vi "6-3 Write.vi"() -> ()   [LabVIEW 2017]
panel:
  out "Waveform Chart":dbl(graph)
  in  "stop":bool
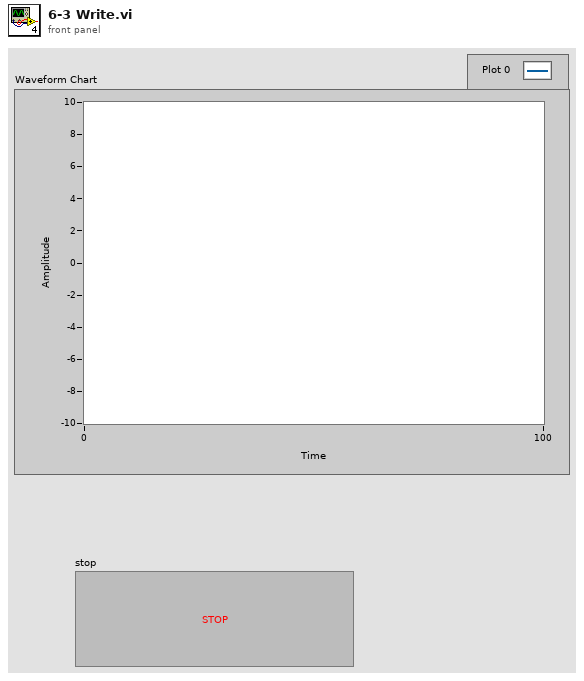
[diagram p1: front panel]
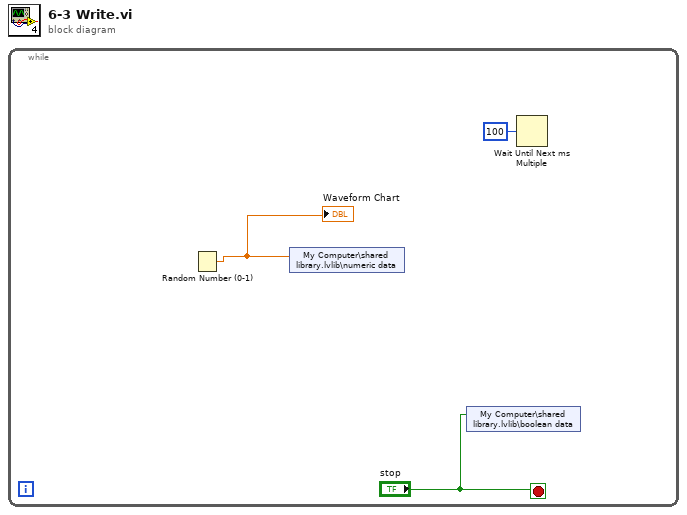
[diagram p0: block diagram]
diagram:
  n1 = while {
    stop <- "stop" stop-if-true
    n2 = Random Number (0-1)() -> (number: 0 to 1=w2:dbl)
    "Waveform Chart" <- w2
    n3 = shared-variable "My Computer\\shared library.lvlib\\numeric data"(w2) -> ()  [unwired: 1 in, 1 out]
    n4 = shared-variable "My Computer\\shared library.lvlib\\boolean data"("stop") -> ()  [unwired: 1 in, 1 out]
    n5 = Wait Until Next ms Multiple(millisecond multiple=u32 100) -> ()  [unwired: 1 out]
  }
